vi "Flatten.vi"(8 "error in":errorcluster, 9 "Data":T1) -> (0 "error out":errorcluster, 2 "Buffer":u8[](array[numeric]) format="%.0x")   [LabVIEW 2020, in "CmdDigitalMultiple.lvlib"]
uses:
  CmdDigitalMultiple.lvlib
  Data.ctl
  CmdDigital/CmdDigital.lvlib
  CmdDigital/Data.ctl
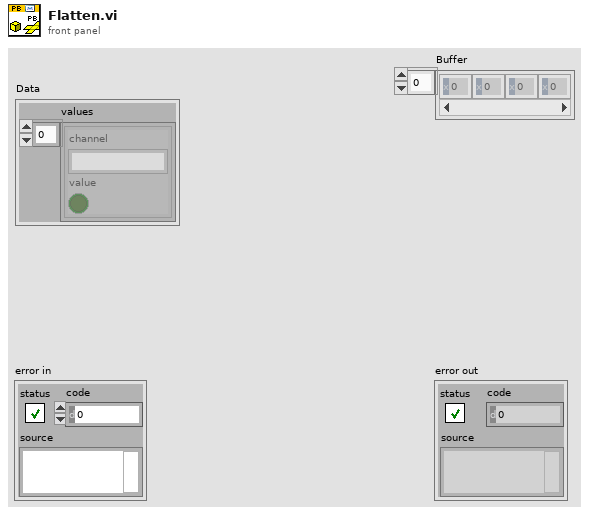
[diagram p1: front panel]
types:
  T1 = typedef "CmdDigitalMultiple.lvlib/Data.ctl" = cluster{"values":T2[]}
  T2 = typedef "CmdDigital.lvlib/Data.ctl" = cluster{"channel":string, "value":bool}
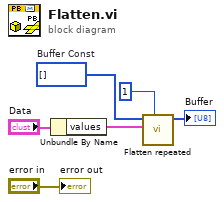
[diagram p0: block diagram]
diagram:
  w4 = u8[] []  # Buffer Const
  n1 = Unbundle By Name("Data") -> ("values"=w3:T2[])
  n2 = call "Flatten repeated.vi"("Field Number"=1, "Data"=w3, "Buffer in"=w4) -> ("Buffer"=→"Buffer":u8[])  [unwired: 8 in]
  "error out" <- "error in"
